vi "Main.vi"() -> ()   [LabVIEW 2020]
uses:
  <vilib>/Utility/config.llb/Read Key (Double).vi
  <vilib>/Utility/config.llb/NI_LVConfig.lvlib
panel:
  out "Status":string
  in  "Abort":bool
  out "Run Time":dbl format="%<%M:%S>t"
  out "LLB":path
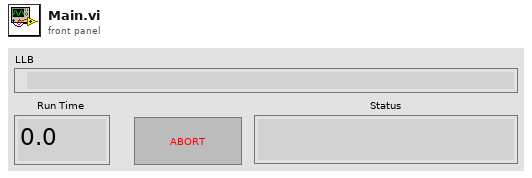
[diagram p1: front panel]
types:
  T1 = cluster{"Overall":dbl, "Categories":cluster{"Category":string, "Value":dbl}[]}
  T2 = typedef "NI_LVConfig.lvlib/Config Data RefNum.ctl" = refnum<k1>
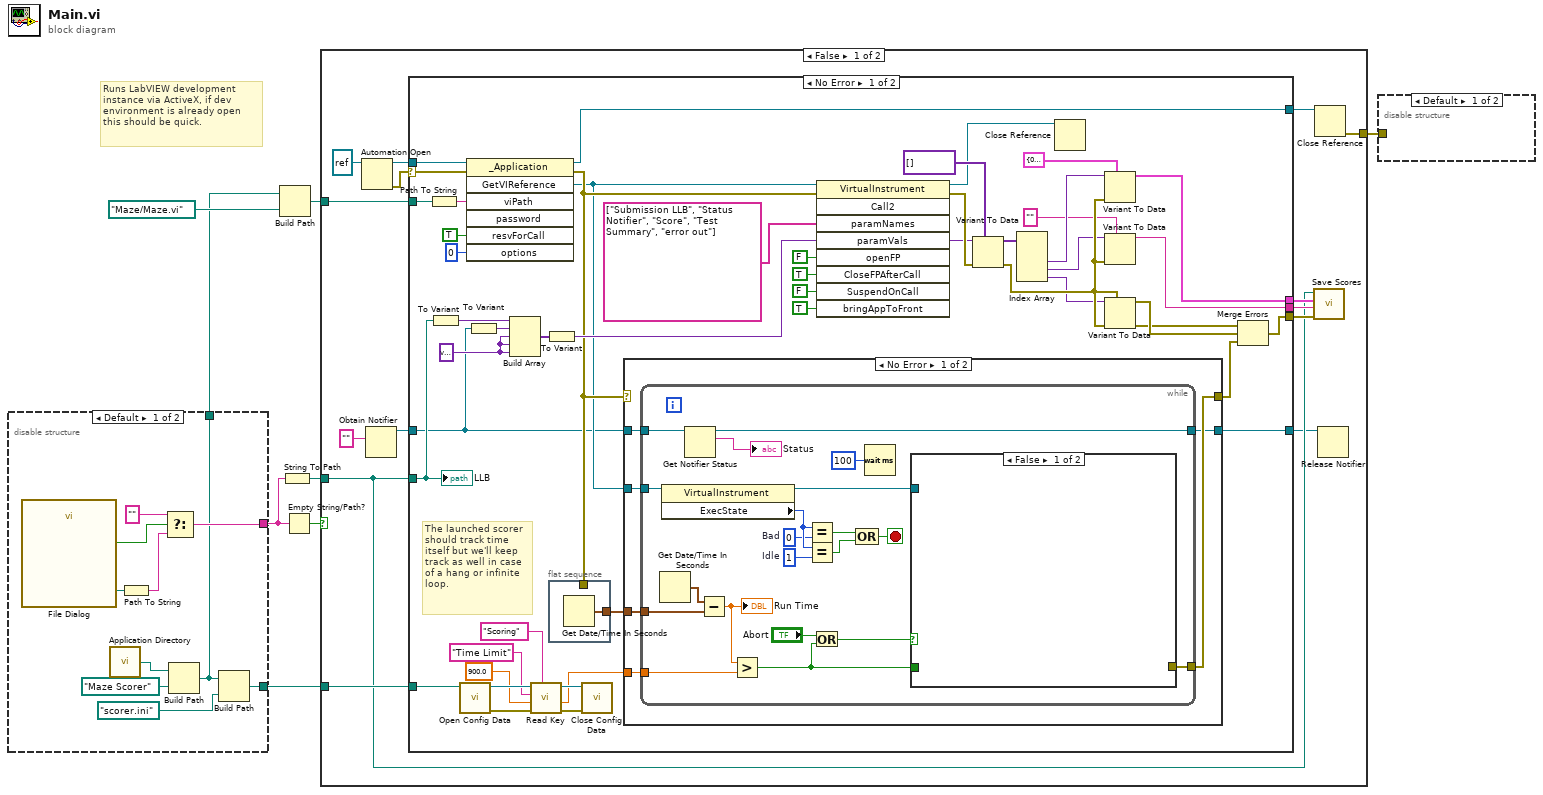
[diagram p0: block diagram]
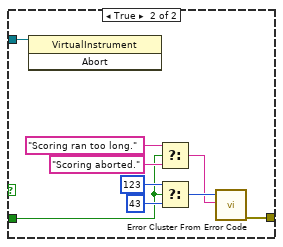
[diagram p2: hidden frame]
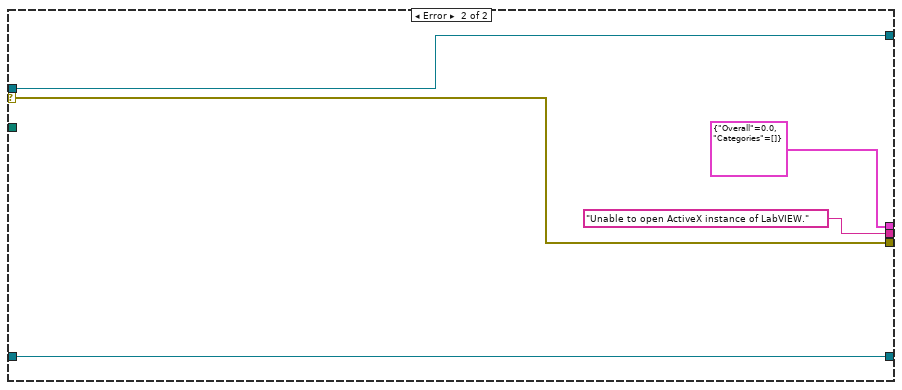
[diagram p4: hidden frame]
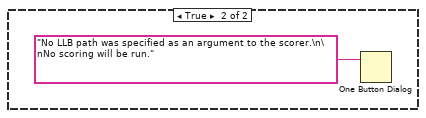
[diagram p5: hidden frame]
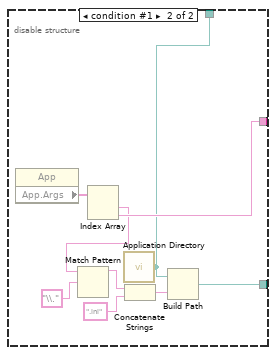
[diagram p6: hidden frame]
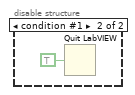
[diagram p7: hidden frame]
diagram:
  # "Runs LabVIEW development instance via ActiveX, if dev environment is already open this should be quick."
  n1 = disable-structure shown="Default" {
    disable-tunnel: [w13 w26] -> w6
    disable-tunnel: [w11 w21] -> w5
    disable-tunnel: [w9 w19] -> w1
    frame condition #0 (active) {
      n2 = call "File Dialog"() -> ("selected path"=w16:path, "cancelled"=w15:bool)  [unwired: 12 in, 2 out]
      n3 = call <vilib>:"Application Directory.vi"() -> ("Application Directory"=w18:path)
      n4 = Path To String(path=w16) -> (string=w14:string)
      n5 = Select(t="", s=w15, f=w14) -> (s? t:f=w13:string)
      n6 = Build Path(base path=w18, name or relative path=path "Maze Scorer") -> (appended path=w9:path)
      n7 = Build Path(base path=w9, name or relative path=path "scorer.ini") -> (appended path=w11:path)
    }
    frame condition #1 {
      n8 = property class="App"() -> ("App.Args"=w27:string[])  [unwired: 2 in, 2 out]
      n9 = Index Array(array=w27) -> (element #1=w20:string, element #2=w26:string)  [unwired: 2 in]
      n10 = Match Pattern(string=w20, regular expression="\\.") -> (before substring=w22:string)  [unwired: 1 in, 3 out]
      n11 = call <vilib>:"Application Directory.vi"() -> ("Application Directory"=w19:path)
      n12 = Concatenate Strings(w22, ".ini" ("string")) -> (w24:string)
      n13 = Build Path(base path=w19, name or relative path=w24) -> (appended path=w21:path)
    }
  }
  n14 = Build Path(base path=w1, name or relative path=path "Maze/Maze.vi") -> (appended path=w3:path)
  n15 = String To Path(string=w6) -> (path=w8:path)
  n16 = Empty String/Path?(string/path=w6) -> (empty?=w7:bool)
  n17 = case shown="False" w7 {
    tunnel: w3 -> [w40 _]
    tunnel: w8 -> [w31 _]
    tunnel: w5 -> [w37 _]
    tunnel: [w33 _] -> w4
    frame False {
      n18 = Automation Open(Automation Refnum=refnum<k7> refnum ("LabVIEW._Application")) -> (Automation Refnum=w32:refnum<k7>, error out=w41:errorcluster)  [unwired: 3 in]
      n19 = Obtain Notifier(notification data type="") -> (notifier out=w29:refnum<notifier>)  [unwired: 3 in, 2 out]
      n20 = case shown="No Error" w41 {
        selector: w41 -> [w87 w130]
        tunnel: w40 -> [w72 _]
        tunnel: [w52 T1 {"Overall"=0.0, "Categories"=[]} ("Score")] -> w39
        tunnel: [w50 "Unable to open ActiveX instance of LabVIEW." ("Test Summary")] -> w38
        tunnel: w31 -> [w69 _]
        tunnel: w37 -> [w77 _]
        tunnel: [w76 w130] -> w36
        tunnel: w32 -> [w74 w133]
        tunnel: [w47 w133] -> w34
        tunnel: w29 -> [w44 w129]
        tunnel: [w42 w129] -> w28
        frame No Error {
          w63 = variant
          # "The launched scorer should track time itself but we'll keep track as well in case of a hang or infinite loop."
          n21 = Path To String(path=w72) -> (string=w71:string)
          n22 = To Variant(anything=w69) -> (Variant=w64:variant)
          n23 = call <vilib>:"Open Config Data.vi"("configuration file path"=w77) -> ("error out"=w84:errorcluster, "refnum"=w85:T2)  [unwired: 8 in, 1 out]
          n24 = invoke class="_Application" method="GetVIReference"(reference=w74, error in=w87, "viPath"=w71, "resvForCall"=TRUE, "options"=0) -> (reference out=w47:refnum<k7>, error out=w46:errorcluster, "GetVIReference"=w45:refnum<k7>)  [unwired: 2 in, 4 out]
          n25 = To Variant(anything=w44) -> (Variant=w43:variant)
          n26 = Build Array(w64, w43, w63, w63, w63) -> (w62:variant[])
          n27 = call-poly <vilib>:"Read Key.vi"("section"="Scoring", "error in (no error)"=w84, "default value"=900.0 ("y"), "key"="Time Limit" ("section"), "refnum"=w85) -> ("error out"=w79:errorcluster, "value"=w78:dbl, "refnum out"=w80:T2)  [unwired: 3 in, 1 out]
          n28 = To Variant(anything=w62) -> (Variant=w60:variant)
          n29 = flat-sequence {
            tunnel: [w91] -> w86
            tunnel: w46 -> [_]
            frame #0 {
              n30 = Get Date/Time In Seconds() -> (seconds since 1Jan1904=w91:timestamp)
            }
          }
          n31 = call <vilib>:"Close Config Data.vi"("error in (no error)"=w79, "refnum"=w80) -> ()  [unwired: 8 in, 2 out]
          n32 = case shown="No Error" w46 {
            selector: w46 -> [_ w128]
            tunnel: w86 -> [w97 _]
            tunnel: w78 -> [w96 _]
            tunnel: [w94 w128] -> w75
            tunnel: w45 -> [w95 _]
            tunnel: w44 -> [w93 w127]
            tunnel: [w92 w127] -> w42
            frame No Error {
              n33 = while {
                tunnel: w97 -> [w117]
                tunnel: w96 -> [w114]
                tunnel: w95 -> [w103]
                tunnel: [w102] -> w94
                tunnel: w93 -> [w100]
                tunnel: [w99] -> w92
                stop <- w112 stop-if-true
                w104 = 1  # Idle
                w105 = 0  # Bad
                n34 = Get Date/Time In Seconds() -> (seconds since 1Jan1904=w116:timestamp)
                n35 = property class="VirtualInstrument"(reference=w103) -> (reference out=w111:refnum<k7>, "ExecState"=w107:i32)  [unwired: 1 in, 1 out]
                n36 = Get Notifier Status(notifier=w100) -> (notifier out=w99:refnum<notifier>, current notification=→"Status":string)  [unwired: 1 in, 3 out]
                n37 = Subtract(x=w116, y=w117) -> (x-y=w115:dbl)
                "Run Time" <- w115
                n38 = Greater?(x=w115, y=w114) -> (0:w108:bool)
                n39 = Equal?(x=w107, y=w105) -> (x = y?=w113:bool)
                n40 = Equal?(x=w107, y=w104) -> (x = y?=w106:bool)
                n41 = Or(x="Abort", y=w108) -> (x .or. y?=w109:bool)
                n42 = Compound Arithmetic op=OR(w113, w106) -> (w112:bool)
                n43 = Wait (ms)(milliseconds to wait=u32 100) -> ()  [unwired: 1 out]
                n44 = case shown="False" w109 {
                  tunnel: w111 -> [_ w119]
                  tunnel: w108 -> [_ w121]
                  tunnel: [_ w118] -> w102
                  frame False {
                  }
                  frame True {
                    n45 = invoke class="VirtualInstrument" method="Abort"(reference=w119) -> ()  [unwired: 2 in, 3 out]
                    n46 = Select(t="Scoring ran too long." ("error message (\"\")"), s=w121, f="Scoring aborted." ("error message (\"\")")) -> (s? t:f=w120:string)
                    n47 = Select(t=123 ("error code (0)"), s=w121, f=43 ("error code (0)")) -> (s? t:f=w124:i32)
                    n48 = call <vilib>:"Error Cluster From Error Code.vi"("error message (\"\")"=w120, "error code (0)"=w124) -> ("error out"=w118:errorcluster)  [unwired: 7 in]
                  }
                }
              }
            }
            frame Error {
            }
          }
          n49 = invoke class="VirtualInstrument" method="Call2"(reference=w45, error in=w46, "paramNames"=string[] ["Submission LLB", "Status Notifier", "Score", "Test Summary", "error out"], "paramVals"=w60, "openFP"=FALSE, "CloseFPAfterCall"=TRUE, "SuspendOnCall"=FALSE, "bringAppToFront"=TRUE) -> (reference out=w48:refnum<k7>, error out=w90:errorcluster, "paramVals"=w59:variant)  [unwired: 1 in, 6 out]
          n50 = Variant To Data(error in=w90, type=variant[] [], Variant=w59) -> (data=w57:variant[], error out=w88:errorcluster)
          n51 = Index Array(array=w57) -> (element #2=w54:variant, element #3=w55:variant, element #4=w56:variant)  [unwired: 4 in, 1 out]
          n52 = Close Reference(reference=w48) -> ()  [unwired: 1 in, 1 out]
          n53 = Variant To Data(error in=w88, type=T1 {"Overall"=0.0, "Categories"=[]} ("Score"), Variant=w54) -> (data=w52:T1)  [unwired: 1 out]
          n54 = Variant To Data(error in=w88, type="", Variant=w55) -> (data=w50:string)  [unwired: 1 out]
          n55 = Variant To Data(error in=w88, type=w88, Variant=w56) -> (data=w89:errorcluster, error out=w49:errorcluster)
          n56 = Merge Errors(w49, w89, w75) -> (w76:errorcluster)
          "LLB" <- w69
        }
        frame Error {
        }
      }
      n57 = call "Save Scores.vi"("error in (no error)"=w36, "Test Summary"=w38, "Score"=w39, "LLB Path"=w31) -> ()  [unwired: 7 in, 1 out]
      n58 = Close Reference(reference=w34) -> (error out=w33:errorcluster)  [unwired: 1 in]
      n59 = Release Notifier(notifier=w28) -> ()  [unwired: 2 in, 3 out]
    }
    frame True {
      n60 = One Button Dialog(message="No LLB path was specified as an argument to the scorer.\n\nNo scoring will be run.") -> ()  [unwired: 1 in, 1 out]
    }
  }
  n61 = disable-structure shown="Default" {
    disable-tunnel: w4 -> [_ _]
    frame condition #0 (active) {
    }
    frame condition #1 {
      n62 = Quit LabVIEW(quit? (T)=TRUE) -> ()
    }
  }
